vi "Event Test.vi"() -> ()   [LabVIEW 2021]
panel:
  out "a":i32
  in  "x":i32
  out "String":string
  in  "Stop 2":bool
  in  "Stop":bool
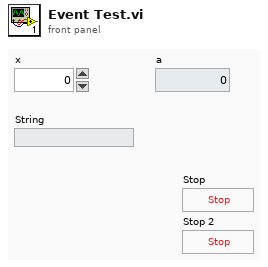
[diagram p1: front panel]
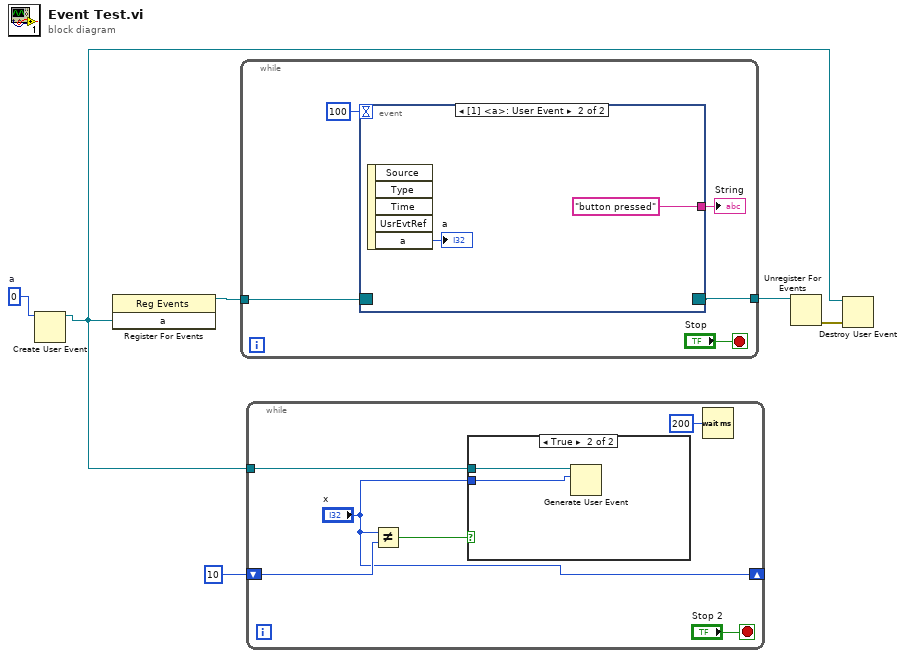
[diagram p0: block diagram]
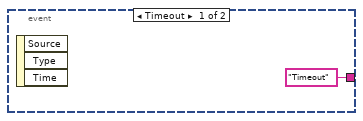
[diagram p3: hidden frame]
diagram:
  w6 = 0  # a
  n1 = Create User Event(user event datatype=w6) -> (user event=w2:refnum<user-event>)  [unwired: 1 in, 1 out]
  n2 = register-events(w2) -> (reference out=w5:refnum<event-registration>)  [unwired: 2 in, 1 out]
  n3 = while {
    tunnel: w5 -> [w10]
    tunnel: [w7] -> w3
    stop <- "Stop" stop-if-true
    n4 = event shown="[1] <a>: User Event" {
      selector: w10 -> [_ _]
      dyn-events: [_ _] -> w7
      timeout: 100 -> [_ _]
      tunnel: ["Timeout" ("String") "button pressed" ("String")] -> w9
      event Timeout {
        n5 = event-data() -> ()  [unwired: 1 in, 3 out]
      }
      event User Event {
        n6 = event-data() -> ("a"=→"a":i32)  [unwired: 1 in, 4 out]
      }
    }
    "String" <- w9
  }
  n7 = while {
    tunnel: w2 -> [w18]
    shift-right: ["x"] -> _
    shift-left: 10 ("event data") -> [w16]
    stop <- "Stop 2" stop-if-true
    n8 = Not Equal?(x="x", y=w16) -> (x != y?=w17:bool)
    n9 = case shown="True" w17 {
      tunnel: w18 -> [_ w22]
      tunnel: "x" -> [_ w21]
      frame False {
      }
      frame True {
        n10 = Generate User Event(user event=w22, event data cluster=w21) -> ()  [unwired: 2 in, 2 out]
      }
    }
    n11 = Wait (ms)(milliseconds to wait=u32 200) -> ()  [unwired: 1 out]
  }
  n12 = Unregister For Events(event registration refnum=w3) -> (error out=w4:errorcluster)  [unwired: 1 in]
  n13 = Destroy User Event(user event=w2, error in=w4) -> ()  [unwired: 1 out]
